vi "SendResponseMessage.vi"(6 "Timeout(ms)":i32, 8 "error in (no error)":errorcluster, 10 "Ack Id":i32, 11 "NetworkConnection in":refnum<class "NetworkConnection.lvclass">) -> (0 "error out":errorcluster, 2 "StillConnected?":bool, 3 "NetworkConnection out":refnum<class "NetworkConnection.lvclass">, 4 "Timed Out?":bool)   [LabVIEW 2023, in "NetworkConnection.lvclass"]
doc: "Writes a message for the Remote System.\n\nJKI Network Streams Connection 1.1.1.15\nJavier Ruiz - JKI\nCopyright (c) 2020, JKI\n\nThis library is provided \"AS IS\" ,WITHOUT WARRANTIES OR CONDITIONS OF ANY KIND, either express or implied."
uses:
  NetworkConnection.lvclass
  NetworkMessage.ctl
  NetworkCommand.ctl
  NetworkConnection.lvclass/NetworkConnection.ctl
  <resource>/objmgr/ni.dex.rc
panel:
  # "Copyright © 2020 JKI All rights reserved.\n\nAuthor: Javier Ruiz <javier.ruiz@jki.net>\n\nThis library is provided \"AS IS\" ,WITHOUT WARRANTIES OR \nCONDITIONS OF ANY KIND, either expressed or implied.\n\nJKI -- jki.net"
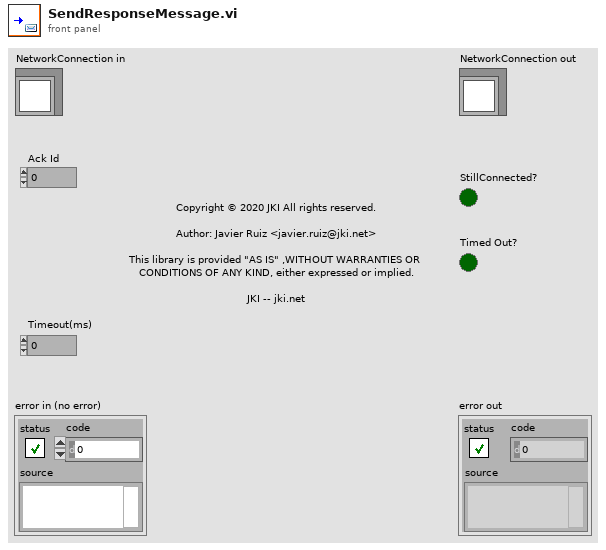
[diagram p1: front panel]
types:
  T1 = typedef "NetworkConnection.lvclass/NetworkMessage.ctl" = cluster{"NetworkCommand":T2, "Wait for Ack?":bool, "Ack Id":i32}
  T2 = typedef "NetworkConnection.lvclass/NetworkCommand.ctl" = cluster{"Message":string, "Message Data":variant}
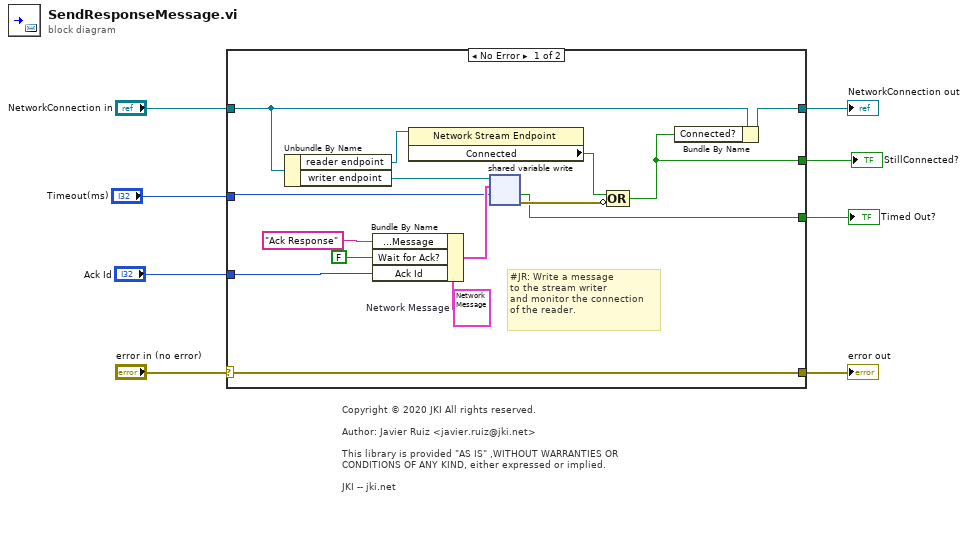
[diagram p0: block diagram]
diagram:
  # "Copyright © 2020 JKI All rights reserved.\n\nAuthor: Javier Ruiz <javier.ruiz@jki.net>\n\nThis library is provided \"AS IS\" ,WITHOUT WARRANTIES OR \nCONDITIONS OF ANY KIND, either expressed or implied.\n\nJKI -- jki.net"
  n1 = case shown="No Error" "error in (no error)" {
    selector: "error in (no error)" -> [w13 w25]
    tunnel: [w13 w25] -> w7
    tunnel: [w14 w24] -> w5
    tunnel: "NetworkConnection in" -> [w21 w24]
    tunnel: "Timeout(ms)" -> [w16 _]
    tunnel: [w15 _] -> w3
    tunnel: [w12 _] -> w2
    tunnel: "Ack Id" -> [w11 _]
    frame No Error {
      w17 = T1 {"NetworkCommand"={"Message"="", "Message Data"=variant}, "Wait for Ack?"=FALSE, "Ack Id"=0}  # Network Message
      # "#JR: Write a message\nto the stream writer\nand monitor the connection\nof the reader."
      n2 = Unbundle By Name(w21) -> ("reader endpoint"=w23:refnum<k21>, "writer endpoint"=w20:refnum<k21>)
      n3 = Bundle By Name(cluster=w17, "NetworkCommand.Message"="Ack Response" ("NetworkCommand.Command"), "Wait for Ack?"=FALSE ("Wait Response?"), "Ack Id"=w11) -> (w18:T1)
      n4 = property class="Network Stream Endpoint"(reference=w23) -> ("Connected"=w22:bool)  [unwired: 1 in, 2 out]
      n5 = shared-variable-write(w20, w18, w16) -> (w19:errorcluster, w12:bool)  [unwired: 1 in, 1 out]
      n6 = Compound Arithmetic op=OR(w22, invert w19) -> (w15:bool)
      n7 = Bundle By Name(cluster=w21, "Connected?"=w15) -> (w14:refnum<class "NetworkConnection.lvclass">)
    }
    frame Error {
    }
  }
  "error out" <- w7
  "NetworkConnection out" <- w5
  "StillConnected?" <- w3
  "Timed Out?" <- w2
